vi "Write Cluster Height.vi"(8 "error in (no error)":errorcluster, 9 "Nested Offsets (None)":cluster{"Label":string, "Offset":i32}[](array[cluster]), 10 "Height":i32, 11 "Cluster in":refnum<vi>) -> (0 "error out":errorcluster, 3 "Cluster":refnum<vi>)   [LabVIEW 2020, in "VolatusGUIEditorCore.lvlib"]
uses:
  VolatusGUIEditorCore.lvlib
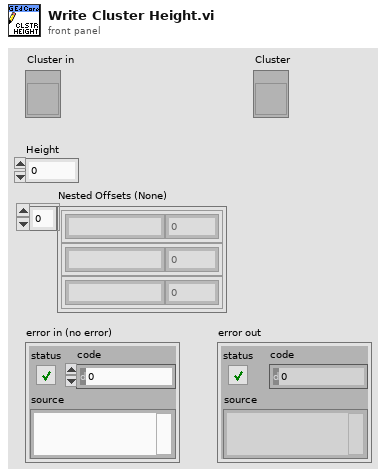
[diagram p1: front panel]
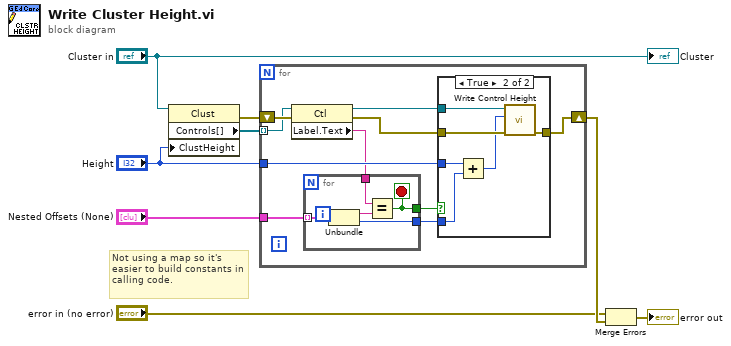
[diagram p0: block diagram]
diagram:
  # "Not using a map so it's easier to build constants in calling code."
  n1 = property class="Clust"(reference="Cluster in", "ClustHeight"="Height") -> (error out=w8:errorcluster, "Controls[]"=w7:refnum<vi>[])  [unwired: 1 in, 1 out]
  n2 = for {
    shift-right: [w9] -> w3
    shift-left: w8 -> [w18]
    tunnel: w7 -> [w17] mode=indexing
    tunnel: "Height" -> [w16]
    tunnel: "Nested Offsets (None)" -> [w15]
    n3 = property class="Ctl"(reference=w17, error in=w18) -> (reference out=w12:refnum<vi>, error out=w10:errorcluster, "Label.Text"=w14:string)
    n4 = for {
      tunnel: w15 -> [w30] mode=indexing
      tunnel: w14 -> [w28]
      tunnel: [w27] -> w13
      tunnel: [w26] -> w11
      stop <- w26 stop-if-true
      n5 = Unbundle(w30) -> ("Label"=w29:string, "Offset"=w27:i32)
      n6 = Equal?(x=w28, y=w29) -> (x = y?=w26:bool)
    }
    n7 = case shown="True" w11 {
      tunnel: w16 -> [_ w24]
      tunnel: w13 -> [_ w23]
      tunnel: w12 -> [_ w22]
      tunnel: w10 -> [w19 w25]
      tunnel: [w19 w20] -> w9
      frame False {
      }
      frame True {
        n8 = Add(x=w24, y=w23) -> (x+y=w21:i32)
        n9 = call "Write Control Height.vi"("error in"=w25, "Height"=w21, "Control in"=w22) -> ("error out"=w20:errorcluster)  [unwired: 7 in, 1 out]
      }
    }
  }
  n10 = Merge Errors("error in (no error)", w3) -> (→"error out":errorcluster)
  "Cluster" <- "Cluster in"
